vi "Error.Update Fault Description.vi"(7 "Append":bool, 10 "New Desc":string, 11 "Default Desc":string) -> (3 "Desc":string)   [LabVIEW 2024, in "EQMF.lvlib" / "Errors.lvlib"]
uses:
  Errors.lvlib
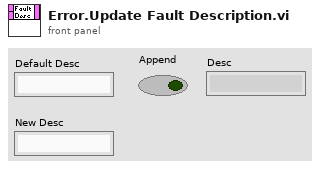
[diagram p1: front panel]
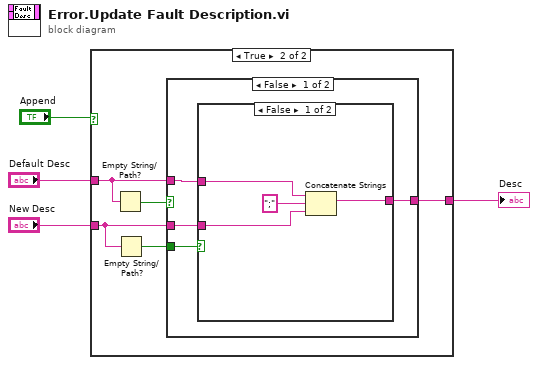
[diagram p0: block diagram]
diagram:
  n1 = case shown="True" "Append" {
    tunnel: "New Desc" -> [w7 w12]
    tunnel: "Default Desc" -> [w6 w13]
    tunnel: [w5 w11] -> w2
    frame False {
      n2 = case shown="Default" w7 {
        selector: w7 -> [_ w9]
        tunnel: w6 -> [w8 _]
        tunnel: [w8 w9] -> w5
        frame "" {
        }
        frame Default {
        }
      }
    }
    frame True {
      n3 = Empty String/Path?(string/path=w13) -> (empty?=w14:bool)
      n4 = Empty String/Path?(string/path=w12) -> (empty?=w10:bool)
      n5 = case shown="False" w14 {
        tunnel: w13 -> [w16 _]
        tunnel: w12 -> [w15 w24]
        tunnel: [w17 w24] -> w11
        tunnel: w10 -> [w18 _]
        frame False {
          n6 = case shown="False" w18 {
            tunnel: [w19 w23] -> w17
            tunnel: w16 -> [w22 w23]
            tunnel: w15 -> [w20 _]
            frame False {
              n7 = Concatenate Strings(w22, ";", w20) -> (w19:string)
            }
            frame True {
            }
          }
        }
        frame True {
        }
      }
    }
  }
  "Desc" <- w2
